vi "Update Load Reference.vi"(8 "error in (no error)":errorcluster, 11 "QControl Creation in":refnum<class "QControl Creation.lvclass">) -> (0 "error out":errorcluster, 3 "QControl Creation (dup)":refnum<class "QControl Creation.lvclass">)   [LabVIEW 2023, in "QControl Creation.lvclass"]
doc: "<b> </b> <b> </b>\n©2016 Q Software Innovations, LLC (QSI)\nwritten by Quentin Alldredge\nproduced in LabVIEW 2015\n\nsupport@qsoftwareinnovations.com\nwww.qsoftwareinnovations.com\n\nAll rights reserved.\n\nRedistribution and use in source and binary forms, with or without modification, are permitted provided that the following conditions are met:\n\n * Redistributions of source code must retain the above copyright notice, this list of conditions and the following disclaimer.\n * Redistributions in binary form must reproduce the above copyright notice, this list of conditions and the following disclaimer in the documentation and/or other materials provided with the distribution.\n * Neither the name of Q Software Innovations, LLC. nor the names of its contributors may be used to endorse or promote products derived from this software without specific prior written permission.\n\nTHIS SOFTWARE IS PROVIDED BY THE COPYRIGHT HOLDERS AND CONTRIBUTORS \"AS IS\" AND ANY EXPRESS OR IMPLIED WARRANTIES, INCLUDING, BUT NOT LIMITED TO, THE IMPLIED WARRANTIES OF MERCHANTABILITY AND FITNESS FOR A PARTICULAR PURPOSE ARE DISCLAIMED. IN NO EVENT SHALL THE COPYRIGHT OWNER OR CONTRIBUTORS BE LIABLE FOR ANY DIRECT, INDIRECT, INCIDENTAL, SPECIAL, EXEMPLARY, OR CONSEQUENTIAL DAMAGES (INCLUDING, BUT NOT LIMITED TO, PROCUREMENT OF SUBSTITUTE GOODS OR SERVICES; LOSS OF USE, DATA, OR PROFITS; OR BUSINESS INTERRUPTION) HOWEVER CAUSED AND ON ANY THEORY OF LIABILITY, WHETHER IN CONTRACT, STRICT LIABILITY, OR TORT (INCLUDING NEGLIGENCE OR OTHERWISE) ARISING IN ANY WAY OUT OF THE USE OF THIS SOFTWARE, EVEN IF ADVISED OF THE POSSIBILITY OF SUCH DAMAGE."
uses:
  QControl Creation.lvclass
  QControl Creation.lvclass/QControl Creation.ctl
  <vilib>/Utility/traverseref.llb/TRef TravTarget.ctl
  <vilib>/Utility/error.llb/Error Cluster From Error Code.vi
  <vilib>/ErrorRing/Error Ring.xnode
  <vilib>/Utility/traverseref.llb/VI Scripting - Traverse.lvlib
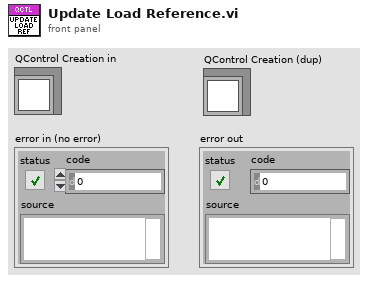
[diagram p1: front panel]
types:
  T1 = typedef "TRef TravTarget.ctl" = enum16{"FP", "BD", "Other"}
  T2 = typedef "ASC_UniqueIDStringParentIDStringName.ctl" = cluster{"Unique ID string":string, "Parent ID string":string, "Class Name (unlocalized)":string, "Class Name (localized)":string}
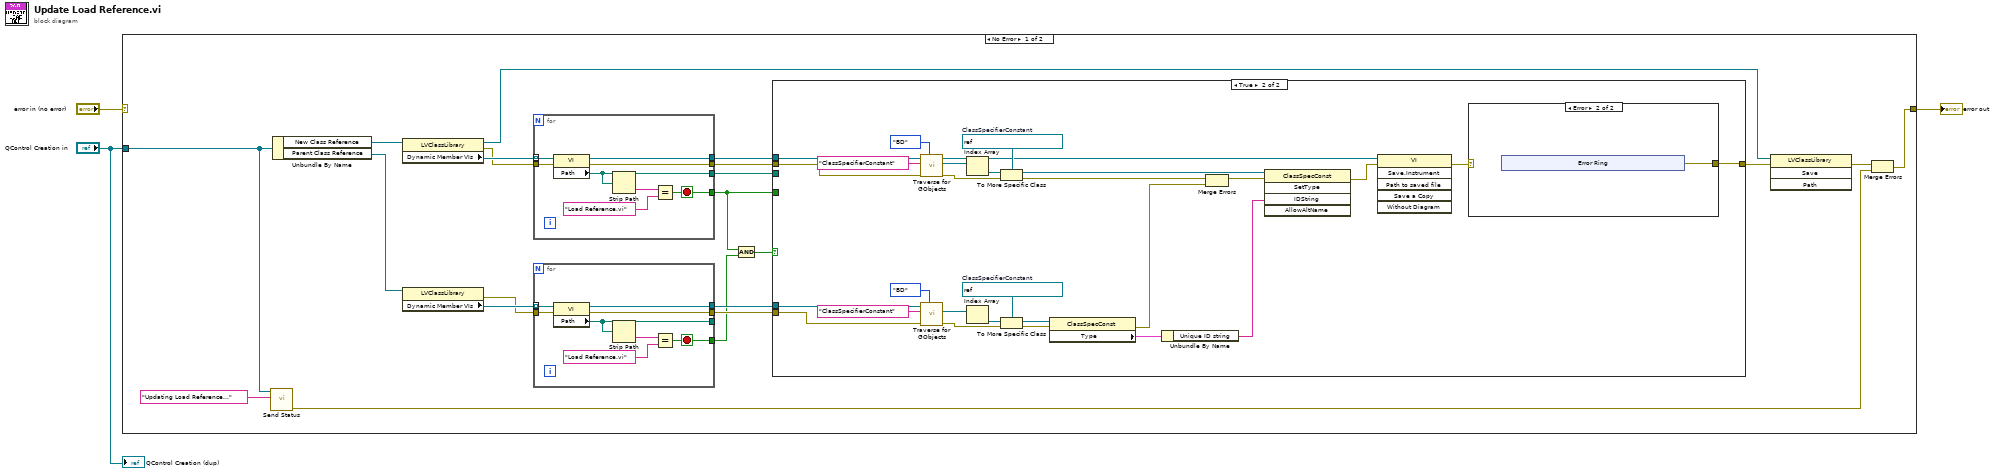
[diagram p0: block diagram]
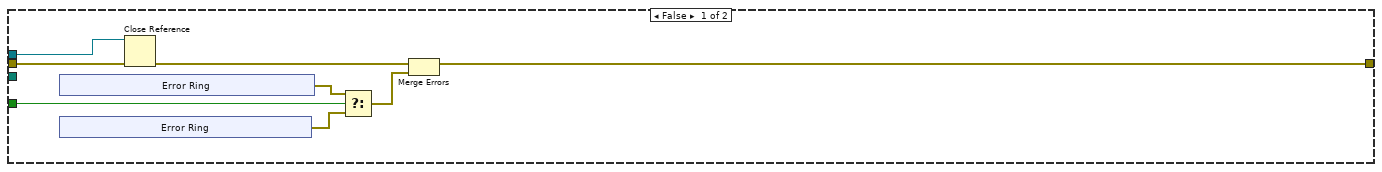
[diagram p2: hidden frame]
diagram:
  n1 = case shown="No Error" "error in (no error)" {
    selector: "error in (no error)" -> [_ w94]
    tunnel: [w5 w94] -> w2
    tunnel: "QControl Creation in" -> [w9 _]
    frame No Error {
      n2 = call "Send Status.vi"("Status"="Updating Load Reference..." ("Value"), "QControl Creation in"=w9) -> ("error out (dup)"=w4:errorcluster)  [unwired: 8 in, 1 out]
      n3 = Unbundle By Name(w9) -> ("New Class Reference"=w22:refnum<vi>, "Parent Class Reference"=w18:refnum<vi>)
      n4 = property class="LVClassLibrary"(reference=w22) -> (reference out=w11:refnum<vi>, error out=w19:errorcluster, "Dynamic Member VIs"=w20:refnum<vi>[])  [unwired: 1 in]
      n5 = property class="LVClassLibrary"(reference=w18) -> (error out=w16:errorcluster, "Dynamic Member VIs"=w17:refnum<vi>[])  [unwired: 1 in, 1 out]
      n6 = for {
        tunnel: w20 -> [w85] mode=indexing
        tunnel: [w80] -> w24
        tunnel: [w79] -> w6
        tunnel: [w78] -> w21
        tunnel: w19 -> [w82]
        tunnel: [w81] -> w23
        stop <- w79 stop-if-true
        n7 = property class="VI"(reference=w85, error in=w82) -> (reference out=w80:refnum<vi>, error out=w81:errorcluster, "Path"=w78:path)
        n8 = Strip Path(path=w78) -> (name=w84:string)  [unwired: 1 out]
        n9 = Equal?(x=w84, y="Load Reference.vi") -> (x = y?=w79:bool)
      }
      n10 = for {
        tunnel: w17 -> [w93] mode=indexing
        tunnel: [w88] -> w15
        tunnel: [w87] -> w7
        tunnel: [w86] -> _
        tunnel: w16 -> [w90]
        tunnel: [w89] -> w14
        stop <- w87 stop-if-true
        n11 = property class="VI"(reference=w93, error in=w90) -> (reference out=w88:refnum<vi>, error out=w89:errorcluster, "Path"=w86:path)
        n12 = Strip Path(path=w86) -> (name=w92:string)  [unwired: 1 out]
        n13 = Equal?(x=w92, y="Load Reference.vi") -> (x = y?=w87:bool)
      }
      n14 = And(x=w6, y=w7) -> (x .and. y?=w8:bool)
      n15 = case shown="True" w8 {
        tunnel: w23 -> [w32 w69]
        tunnel: [w31 w44] -> w13
        tunnel: w24 -> [w29 w70]
        tunnel: w21 -> [_ _]
        tunnel: w15 -> [_ w53]
        tunnel: w14 -> [_ w52]
        tunnel: w6 -> [w28 _]
        frame False {
          n16 = xnode "Error Ring"() -> ("error out"=w25:errorcluster)
          n17 = xnode "Error Ring"() -> ("error out"=w27:errorcluster)
          n18 = Close Reference(reference=w29, error in (no error)=w32) -> (error out=w30:errorcluster)
          n19 = Select(t=w25, s=w28, f=w27) -> (s? t:f=w26:errorcluster)
          n20 = Merge Errors(w30, w26) -> (w31:errorcluster)
        }
        frame True {
          w59 = refnum<vi> refnum  # ClassSpecifierConstant
          w63 = refnum<vi> refnum  # ClassSpecifierConstant
          n21 = call <vilib>:"Traverse for GObjects.vi"("Traverse Target"=TRef_TravTarget."BD", "error in (no error)"=w69, "Class Name"="ClassSpecifierConstant", "VI Refnum"=w70) -> ("error out"=w64:errorcluster, "References"=w66:refnum<vi>[], "dup VI Refnum"=w60:refnum<vi>)  [unwired: 4 in, 1 out]
          n22 = call <vilib>:"Traverse for GObjects.vi"("Traverse Target"=TRef_TravTarget."BD", "error in (no error)"=w52, "Class Name"="ClassSpecifierConstant", "VI Refnum"=w53) -> ("error out"=w58:errorcluster, "References"=w56:refnum<vi>[])  [unwired: 4 in, 2 out]
          n23 = Index Array(array=w66) -> (element=w65:refnum<vi>)  [unwired: 1 in]
          n24 = Index Array(array=w56) -> (element=w57:refnum<vi>)  [unwired: 1 in]
          n25 = To More Specific Class(target class=w63, reference=w65, error in=w64) -> (specific class reference=w62:refnum<vi>, error out=w61:errorcluster)
          n26 = To More Specific Class(target class=w59, reference=w57, error in=w58) -> (specific class reference=w51:refnum<vi>, error out=w45:errorcluster)
          n27 = property class="ClassSpecConst"(reference=w51, error in=w45) -> (error out=w46:errorcluster, "Type"=w50:T2)  [unwired: 1 out]
          n28 = Unbundle By Name(w50) -> ("Unique ID string"=w49:string)
          n29 = Merge Errors(w61, w46) -> (w47:errorcluster)
          n30 = invoke class="ClassSpecConst" method="SetType"(reference=w62, error in=w47, "IDString"=w49) -> (error out=w48:errorcluster)  [unwired: 2 in, 4 out]
          n31 = invoke class="VI" method="Save.Instrument"(reference=w60, error in=w48) -> (error out=w43:errorcluster)  [unwired: 4 in, 5 out]
          n32 = case shown="Error" w43 {
            selector: w43 -> [w71 _]
            tunnel: [w71 w72] -> w44
            frame No Error {
            }
            frame Error {
              n33 = xnode "Error Ring"() -> ("error out"=w72:errorcluster)
            }
          }
        }
      }
      n34 = invoke class="LVClassLibrary" method="Save"(reference=w11, error in=w13) -> (error out=w12:errorcluster)  [unwired: 2 in, 3 out]
      n35 = Merge Errors(w12, w4) -> (w5:errorcluster)
    }
    frame Error {
    }
  }
  "error out" <- w2
  "QControl Creation (dup)" <- "QControl Creation in"
